vi "Falg sync test.vi"() -> ()   [LabVIEW 2015]
panel:
  out "Array 3":bool[](array[boolean])
  out "Array 2":bool[](array[boolean])
  in  "Array":bool[](array[boolean])=[FALSE, TRUE, TRUE, FALSE, FALSE, FALSE, FALSE, FALSE]
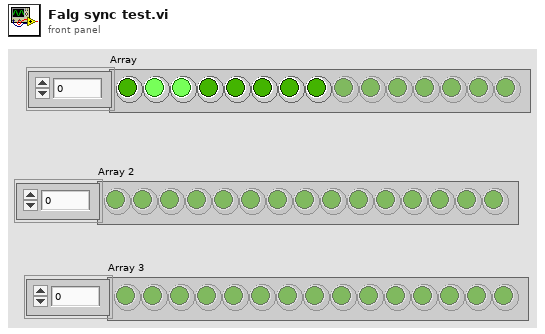
[diagram p1: front panel]
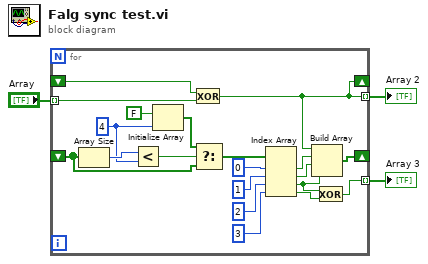
[diagram p0: block diagram]
diagram:
  n1 = for {
    shift-right: [w19] -> _
    shift-left: _ -> [w23]
    tunnel: "Array" -> [w22] mode=indexing
    tunnel: [w19] -> w2 mode=indexing
    shift-right: [w20] -> _
    shift-left: _ -> [w12]
    tunnel: [w7] -> w1 mode=indexing
    w16 = 4 ("y")
    n2 = Array Size(array=w12) -> (size(s)=w17:i32)
    n3 = Less?(x=w17, y=w16) -> (x < y?=w14:bool)
    n4 = Initialize Array(FALSE, w16) -> (w13:bool[])
    n5 = Exclusive Or(1:w22, 2:w23) -> (0:w19:bool)
    n6 = Select(t=w13, s=w14, f=w12) -> (s? t:f=w11:bool[])
    n7 = Index Array(array=w11, index #1=0 ("index"), index #2=1 ("index"), index #3=2 ("index"), index #4=3 ("index")) -> (element #1=w21:bool, element #2=w8:bool, element #3=w4:bool, element #4=w5:bool)
    n8 = Build Array(w19, w21, w8, w4) -> (w20:bool[])
    n9 = Exclusive Or(1:w5, 2:w4) -> (0:w7:bool)
  }
  "Array 2" <- w2
  "Array 3" <- w1
